vi "Set_RegData_Value.vi"(8 "error in (no error)":errorcluster, 10 "New Val":string, 11 "RegData_I32 in":refnum<class "IB_RegData_I32.lvclass">) -> (0 "error out":errorcluster, 2 "Val":string, 3 "RegData_I32 out":refnum<class "IB_RegData_I32.lvclass">)   [LabVIEW 2020, in "IB_RegData_I32.lvclass"]
uses:
  <vilib>/AppBuilder/IB_Classes/RegData/RegData_I32/IB_RegData_I32.lvclass
  <vilib>/AppBuilder/IB_Classes/RegData/RegData_I32/IB_RegData_I32.lvclass/IB_RegData_I32.ctl
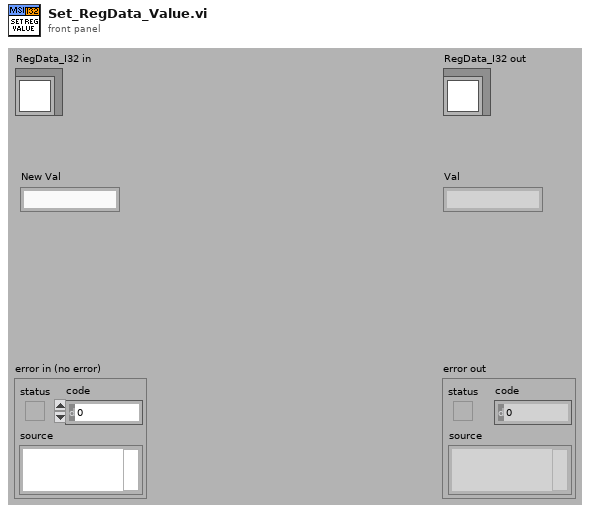
[diagram p1: front panel]
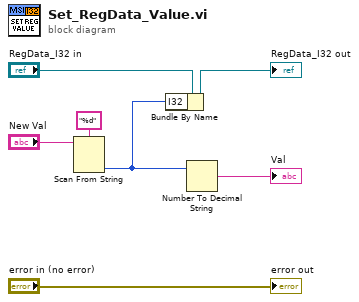
[diagram p0: block diagram]
diagram:
  n1 = Scan From String(format string="%d", input string="New Val") -> (output 1=w2:i32)  [unwired: 2 in, 4 out]
  n2 = Bundle By Name(cluster="RegData_I32 in", "I32"=w2) -> (→"RegData_I32 out":refnum<class "IB_RegData_I32.lvclass">)
  n3 = Number To Decimal String(number=w2) -> (decimal integer string=→"Val":string)  [unwired: 1 out]
  "error out" <- "error in (no error)"
